vi "Read Configuration to gRPC.vi"(8 "error in (no error)":errorcluster, 11 "CIFPlugin in":refnum<class "Template_Plugin.lvclass">) -> (0 "error out":errorcluster, 2 "Configuration":T1={"Common"={"Period (s)"=0.001, "Offset (us)"=0, "Priority"=100, "Processor"=-2, "External Clock"={"ClockID"=0, "Clock Name"="", "Publish Clock"=FALSE, "Convert Data Timestamps"=FALSE, "Plugin Timing Source"=FALSE}}, "Step"=100} {"Common"."Period (s)" format="%#_13g"}, 3 "CIFPlugin out":refnum<class "Template_Plugin.lvclass">)   [LabVIEW 2021, in "Template_Plugin.lvclass"]
doc: "Updates to the configuration will not be automatically updated in the custom gRPC loop. To get the latest configuration the DVR used to pass configuration data from the core gRPC loop to the main loop can be read directly."
uses:
  Template_Plugin.lvclass
  C:/Program Files/National Instruments/LabVIEW 2021/vi.lib/CIF Foundation/CIF Core/CIFCore/Class/CIFCorePlugin.lvclass
  Common/Typedef/Configuration.ctl
  <vilib>/CIF Foundation/CIF Core/CIFCore/Common/Typedef/Common Plugin Configuration.ctl
  <vilib>/CIF Foundation/CIF Core/CIFCore/Common/Typedef/External Clock Config.ctl
  Template_Plugin.lvclass/Template_Plugin.ctl
  <vilib>/CIF Foundation/CIF Core/CIFCore/Class/CIFCorePlugin.lvclass
  <vilib>/CIF Foundation/CIF Core/CIFCore/Common/CIFCoreCommon.lvlib
  Common/Template_Common.lvlib
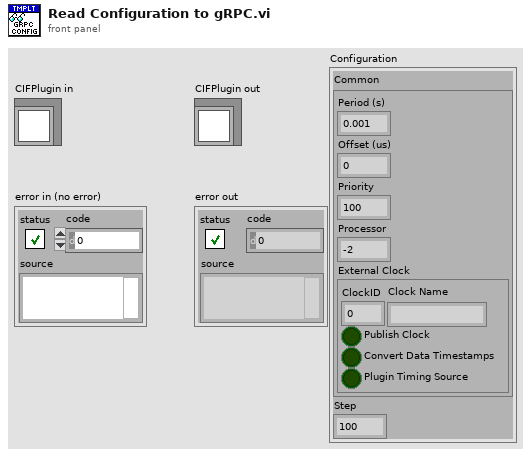
[diagram p1: front panel]
types:
  T1 = typedef "Template_Common.lvlib/Configuration.ctl" = cluster{"Common":T2, "Step":u64}
  T2 = typedef "CIFCoreCommon.lvlib/Common Plugin Configuration.ctl" = cluster{"Period (s)":dbl, "Offset (us)":i32, "Priority":i32, "Processor":i32, "External Clock":T3}
  T3 = typedef "CIFCoreCommon.lvlib/External Clock Config.ctl" = cluster{"ClockID":u8, "Clock Name":string, "Publish Clock":bool, "Convert Data Timestamps":bool, "Plugin Timing Source":bool}
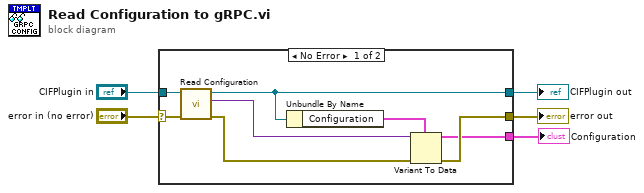
[diagram p0: block diagram]
diagram:
  n1 = case shown="No Error" "error in (no error)" {
    selector: "error in (no error)" -> [w12 w14]
    tunnel: "CIFPlugin in" -> [w13 w15]
    tunnel: [w7 w15] -> w2
    tunnel: [w8 w14] -> w4
    tunnel: [w6 _] -> w1
    frame No Error {
      n2 = call <vilib>:"Read Configuration.vi"("error in"=w12, "CIFCorePlugin in"=w13) -> ("error out"=w11:errorcluster, "Configuration Data"=w10:variant, "CIFCorePlugin out"=w7:refnum<class "Template_Plugin.lvclass">)  [unwired: 7 in]
      n3 = Unbundle By Name(w7) -> ("Configuration"=w9:T1)
      n4 = Variant To Data(error in=w11, type=w9, Variant=w10) -> (data=w6:T1, error out=w8:errorcluster)
    }
    frame Error {
    }
  }
  "error out" <- w4
  "CIFPlugin out" <- w2
  "Configuration" <- w1
